vi "Get Audio Settings.vi"(8 "error in (no error)":errorcluster) -> (0 "error out":errorcluster, 3 "audio settings":T1)   [LabVIEW 2022 SP3, in "Config Dialog.lvlib"]
uses:
  Config Dialog.lvlib
  audio settings.ctl
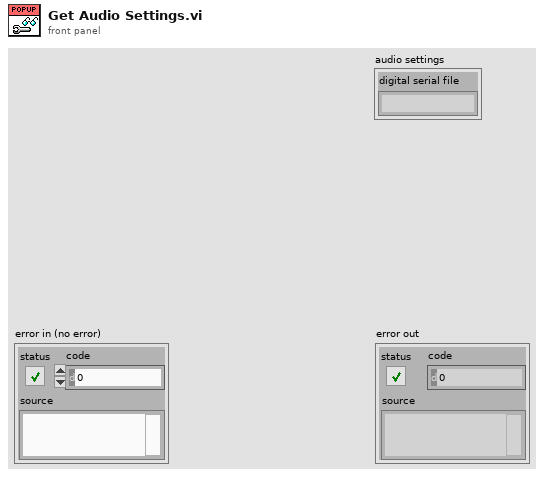
[diagram p1: front panel]
types:
  T1 = typedef "Config Dialog.lvlib/audio settings.ctl" = cluster{"digital serial file":string}
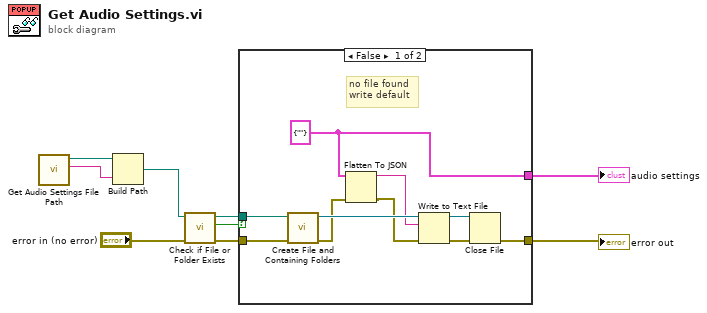
[diagram p0: block diagram]
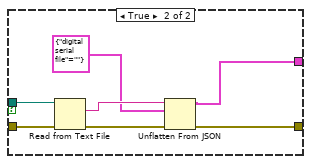
[diagram p2: hidden frame]
diagram:
  n1 = call "Get Audio Settings File Path.vi"() -> ("file name"=w4:string, "directory"=w5:path)  [unwired: 10 in]
  n2 = Build Path(base path=w5, name or relative path=w4) -> (appended path=w3:path)
  n3 = call <vilib>:"Check if File or Folder Exists.vi"("error in (no error)"="error in (no error)", "path"=w3) -> ("error out"=w9:errorcluster, "file or folder exists?"=w8:bool, "dup path"=w7:path)  [unwired: 7 in]
  n4 = case shown="False" w8 {
    tunnel: w9 -> [w19 w25]
    tunnel: w7 -> [w18 w26]
    tunnel: [w15 w21] -> w2
    tunnel: [w12 w20] -> w1
    frame False {
      w12 = T1 {"digital serial file"=""} ("audio settings")
      # "no file found\nwrite default"
      n5 = call <vilib>:"Create File and Containing Folders.vi"("error in (no error)"=w19, "file path"=w18) -> ("error out"=w13:errorcluster, "refnum out"=w14:refnum<file>)  [unwired: 8 in]
      n6 = Flatten To JSON(anything=w12, error in (no error)=w13) -> (JSON string=w10:string, 11:w11:errorcluster)  [unwired: 1 in]
      n7 = Write to Text File(file (use dialog)=w14, text=w10, error in=w11) -> (refnum out=w16:refnum<file>, error out=w17:errorcluster)  [unwired: 1 in, 1 out]
      n8 = Close File(refnum=w16, error in=w17) -> (error out=w15:errorcluster)  [unwired: 1 out]
    }
    frame True {
      n9 = Read from Text File(file (use dialog)=w26, error in=w25) -> (text=w23:string, error out=w24:errorcluster)  [unwired: 2 in, 2 out]
      n10 = Unflatten From JSON(JSON string=w23, type and defaults=T1 {"digital serial file"=""} ("audio settings"), error in (no error)=w24) -> (value=w20:T1, error out=w21:errorcluster)  [unwired: 4 in]
    }
  }
  "error out" <- w2
  "audio settings" <- w1
